vi "Do.vi"(8 "error in (no error)":errorcluster, 10 "Actor in":refnum<class "Actor.lvclass">, 11 "GetRecord Msg":refnum<class "GetRecord Msg.lvclass">) -> (0 "error out":errorcluster, 2 "Actor out":refnum<class "Actor.lvclass">)   [LabVIEW 2025, in "DAQ_Module.lvlib" / "GetRecord Msg.lvclass"]
doc: "This VI delivers the message to the actor by calling the appropriate method(s) on the actor."
uses:
  GetRecord Msg.lvclass
  <vilib>/ActorFramework/Actor/Actor.lvclass
  GetRecord Msg.lvclass/GetRecord Msg.ctl
  DAQ_Module/DAQ_Module.lvclass
  C:/Program Files (x86)/National Instruments/LabVIEW 2025/vi.lib/ActorFramework/Actor/Actor.lvclass
  9ef47adc-f318-494c-9b8b-6df3216d6863.vi
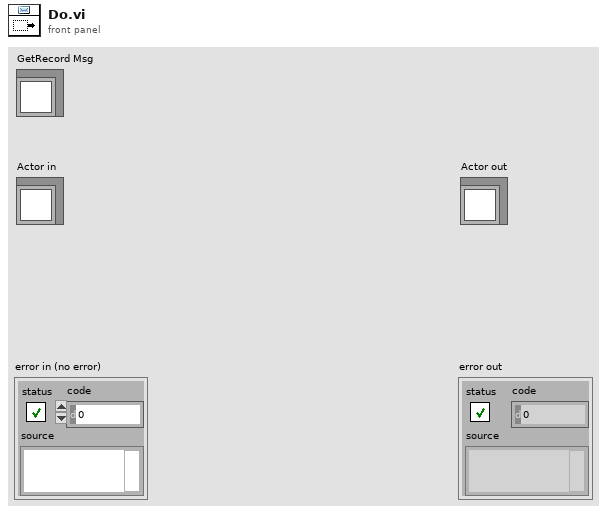
[diagram p1: front panel]
types:
  T1 = typedef "Task_Abstr.lvlib/Task_Abstr.lvclass/WaveformData.ctl" = cluster{"StartTime":timestamp, "StopTime":timestamp, "Waveform":waveform(dbl)[]}
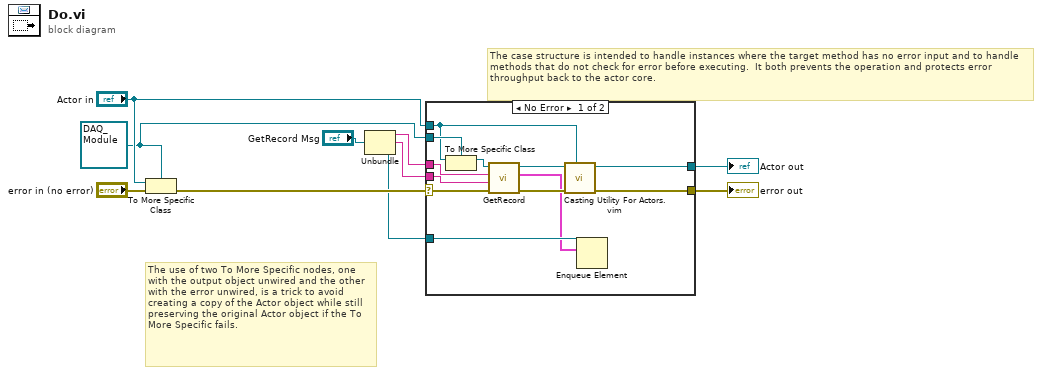
[diagram p0: block diagram]
diagram:
  w4 = refnum<class "DAQ_Module.lvclass"> refnum ("Actor in")
  # "The use of two To More Specific nodes, one with the output object unwired and the other with the error unwired, is a trick to avoid creating a copy of the Actor object while still preserving the original Actor object if the To More Specific fails."
  # "The case structure is intended to handle instances where the target method has no error input and to handle methods that do not check for error before executing.  It both prevents the operation and protects error throughput back to the actor core."
  n1 = To More Specific Class(target class=w4, reference="Actor in", error in="error in (no error)") -> (error out=w8:errorcluster)  [unwired: 1 out]
  n2 = Unbundle("GetRecord Msg") -> (w3:string, w2:string, w1:refnum<queue>)
  n3 = case shown="No Error" w8 {
    selector: w8 -> [w22 w24]
    tunnel: [w16 w24] -> w7
    tunnel: [w17 w23] -> w6
    tunnel: "Actor in" -> [w19 w23]
    tunnel: w4 -> [w20 _]
    tunnel: w3 -> [w14 _]
    tunnel: w2 -> [w13 _]
    tunnel: w1 -> [w12 _]
    frame No Error {
      n4 = To More Specific Class(target class=w20, reference=w19) -> (specific class reference=w21:refnum<class "DAQ_Module.lvclass">)  [unwired: 1 in, 1 out]
      n5 = call "GetRecord.vi"("error in (no error)"=w22, "Label"=w13, "Task"=w14, "DAQ_Module in"=w21) -> ("error out"=w15:errorcluster, "RecordData"=w11:T1, "DAQ_Module out"=w18:refnum<class "DAQ_Module.lvclass">)  [unwired: 5 in]
      n6 = call "Casting Utility For Actors.vim"("type"=w19, "error in (no error)"=w15, "Actor in"=w18) -> ("error out"=w16:errorcluster, "Actor out"=w17:refnum<class "Actor.lvclass">)  [unwired: 7 in]
      n7 = Enqueue Element(queue=w12, element=w11) -> ()  [unwired: 2 in, 3 out]
    }
    frame Error {
      # "If type check fails, pass the original object out again."
    }
  }
  "error out" <- w7
  "Actor out" <- w6
